vi "DC(P+V)_3Wheel.vi"(8 "CMD":cluster{"Tcmd":dbl, "Ocmd":dbl, "itrflg":i32}, 11 "control":T1) -> (0 "output cluster 2":cluster{"LPerr":dbl}, 3 "output cluster":T1)   [LabVIEW 2013]
uses:
  Global.vi
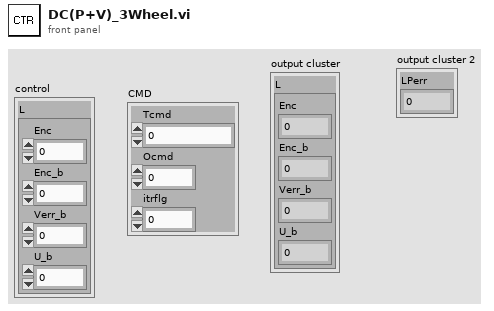
[diagram p1: front panel]
types:
  T1 = cluster{"L":cluster{"Enc":dbl, "Enc_b":dbl, "Verr_b":dbl, "U_b":dbl}}
  T2 = cluster{"Kvff":dbl, "Kpp":dbl, "Kvp":dbl, "Kvi":dbl, "Friction":dbl}
  T3 = typedef "DC Motor Port.ctl" = u16
  T4 = cluster{"MM2DEG":dbl, "PLS2DEG":dbl, "Ts":dbl, "Tcnt":i32, "fs":i32, "Vmax":dbl, "Jmax":dbl, "N_Delay":i32, "C_port":T3, "KNRPLS":dbl}
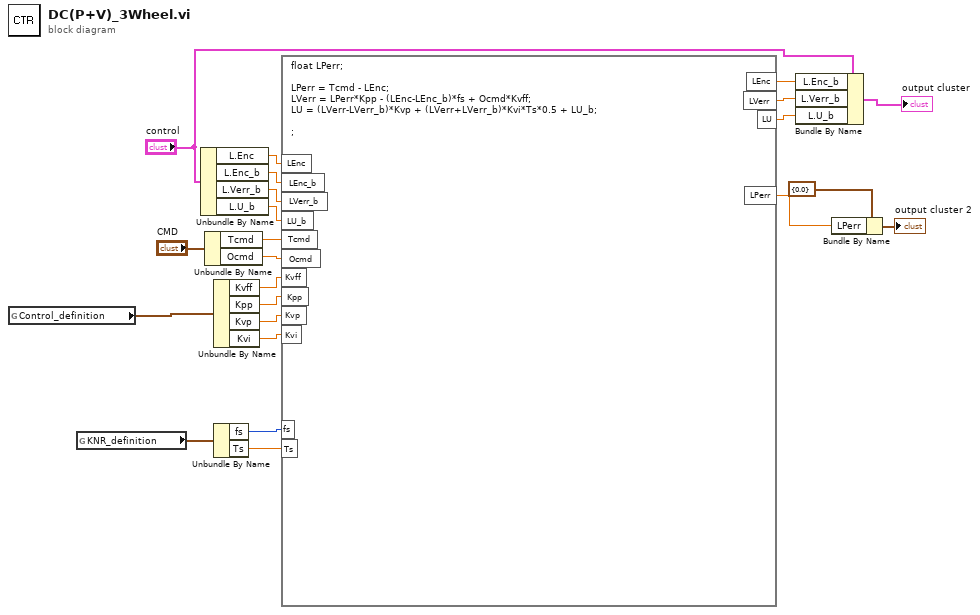
[diagram p0: block diagram]
diagram:
  n1 = global read "Global.vi" "Control_definition"() -> (w15:T2)
  n2 = global read "Global.vi" "KNR_definition"() -> (w8:T4)
  n3 = Unbundle By Name("control") -> ("L.Enc"=w10:dbl, "L.Enc_b"=w9:dbl, "L.Verr_b"=w6:dbl, "L.U_b"=w4:dbl)
  n4 = Unbundle By Name("CMD") -> ("Tcmd"=w23:dbl, "Ocmd"=w22:dbl)
  n5 = Unbundle By Name(w15) -> ("Kvff"=w14:dbl, "Kpp"=w13:dbl, "Kvp"=w12:dbl, "Kvi"=w11:dbl)
  n6 = Unbundle By Name(w8) -> ("fs"=w7:i32, "Ts"=w5:dbl)
  n7 = formula code="float LPerr;\n\nLPerr = Tcmd - LEnc;\nLVerr = LPerr*Kpp - (LEnc-LEnc_b)*fs + Ocmd*Kvff;\nLU = (LVerr-LVerr_b)*Kvp + (LVerr+LVerr_b)*Kvi*Ts*0.5 + LU_b;\n\n;"("Tcmd"=w23, "Ocmd"=w22, "LEnc"=w10, "LEnc_b"=w9, "LVerr_b"=w6, "LU_b"=w4, "Kvff"=w14, "Kpp"=w13, "Kvp"=w12, "Kvi"=w11, "fs"=w7, "Ts"=w5) -> ("LVerr"=w19:dbl, "LU"=w18:dbl, "LPerr"=w16:dbl, "LEnc"=w20:dbl)
  n8 = Bundle By Name(cluster="control", "L.Enc_b"=w20, "L.Verr_b"=w19, "L.U_b"=w18) -> (→"output cluster":T1)
  n9 = Bundle By Name(cluster=cluster{"LPerr":dbl} {"LPerr"=0.0} ("Cluster"), "LPerr"=w16) -> (→"output cluster 2":cluster{"LPerr":dbl})
